vi "Check_Frame_Continuity.vi"(2 "N":u32) -> (0 "Missing Frames":u32[](array[numeric]), 1 "No of missed frames":i32)   [LabVIEW 2015]
panel:
  in  "Track Of Missing Frames":u32[](array[numeric])
  in  "N-1":u32
  # "PERFORMANCE UNKNOWN"
  # "OUTPUT"
  # "INPUT"
  # "Internal Variables"
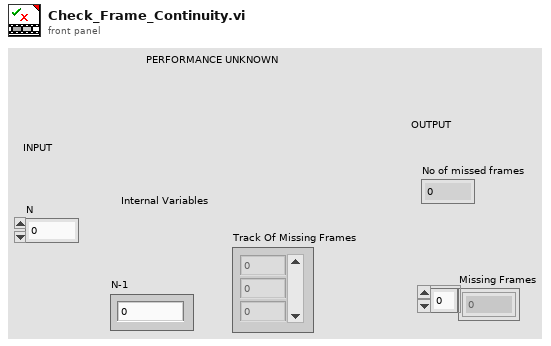
[diagram p1: front panel]
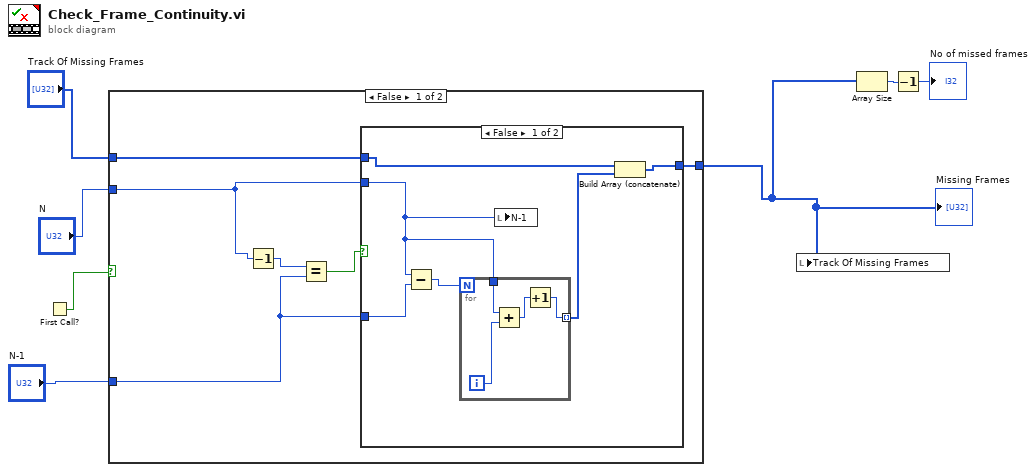
[diagram p0: block diagram]
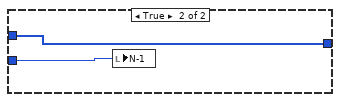
[diagram p2: hidden frame]
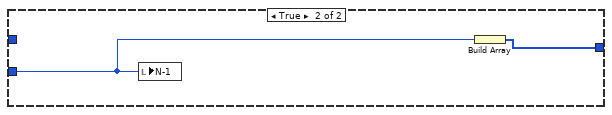
[diagram p3: hidden frame]
diagram:
  n1 = First Call?() -> (First Call?: T/F=w4:bool)
  n2 = case shown="False" w4 {
    tunnel: "N-1" -> [w8 _]
    tunnel: "N" -> [w11 w26]
    tunnel: "Track Of Missing Frames" -> [w10 _]
    tunnel: [w9 w27] -> w3
    frame False {
      n3 = Decrement(x=w11) -> (x-1=w13:u32)
      n4 = Equal?(x=w13, y=w8) -> (x = y?=w12:bool)
      n5 = case shown="False" w12 {
        tunnel: w11 -> [w14 w25]
        tunnel: w10 -> [w16 w24]
        tunnel: [w17 w24] -> w9
        tunnel: w8 -> [w19 _]
        frame False {
          n6 = Subtract(x=w14, y=w19) -> (x-y=w18:u32)
          n7 = for {
            N: w18 -> [_]
            tunnel: w14 -> [w23]
            tunnel: [w21] -> w15 mode=indexing
            i -> [w22]
            n8 = Add(x=w23, y=w22) -> (x+y=w20:u32)
            n9 = Increment(x=w20) -> (x+1=w21:u32)
          }
          n10 = local write "N-1"(w14) -> ()
          n11 = Build Array (concatenate)(w16, w15) -> (w17:u32[])
        }
        frame True {
          n12 = local write "N-1"(w25) -> ()
        }
      }
    }
    frame True {
      n13 = local write "N-1"(w26) -> ()
      n14 = Build Array(w26) -> (w27:u32[])
    }
  }
  "Missing Frames" <- w3
  n15 = local write "Track Of Missing Frames"(w3) -> ()
  n16 = Array Size(array=w3) -> (size(s)=w1:i32)
  n17 = Decrement(x=w1) -> (x-1=→"No of missed frames":i32)
